vi "Load and Save Example.vi"() -> ()   [LabVIEW 2015]
uses:
  poly_persist_controls_auto_read.vi
  core_persist_controls_auto.vi
  poly_persist_controls_auto_write.vi
panel:
  in  "Cancel":bool
  in  "OK":bool
  in  "Numeric Option 2":dbl
  in  "Numeric Option 1":dbl
  in  "Option 4":bool
  in  "Option 3":bool
  in  "Option 2":bool
  in  "Option 1":bool
  in  "User":u16(ring) items=["John", "Paul", "George", "Ringo"]
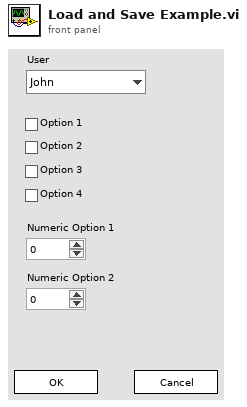
[diagram p1: front panel]
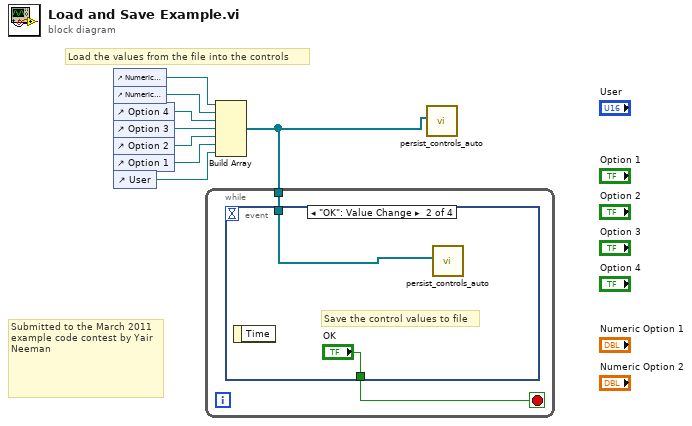
[diagram p0: block diagram]
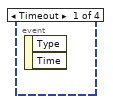
[diagram p2: hidden frame]
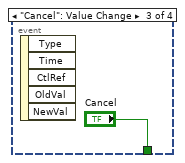
[diagram p3: hidden frame]
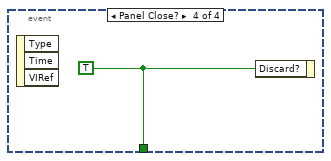
[diagram p4: hidden frame]
diagram:
  # "Submitted to the March 2011 example code contest by Yair Neeman"
  # "Load the values from the file into the controls"
  n1 = control-ref of="Numeric Option 2"() -> (w8:refnum<vi>)
  n2 = control-ref of="Numeric Option 1"() -> (w7:refnum<vi>)
  n3 = control-ref of="Option 4"() -> (w6:refnum<vi>)
  n4 = control-ref of="Option 3"() -> (w5:refnum<vi>)
  n5 = control-ref of="Option 2"() -> (w4:refnum<vi>)
  n6 = control-ref of="Option 1"() -> (w3:refnum<vi>)
  n7 = control-ref of="User"() -> (w2:refnum<vi>)
  n8 = Build Array(w8, w7, w6, w5, w4, w3, w2) -> (w1:refnum<vi>[])
  n9 = while {
    tunnel: w1 -> [w9]
    stop <- w10 stop-if-true
    n10 = event shown="[1] \"OK\": Value Change" {
      selector: _ -> [_ _ _ _]
      dyn-events: _ -> [_ _ _ _]
      timeout: _ -> [_ _ _ _]
      tunnel: [_ "OK" "Cancel" w14] -> w10
      tunnel: w9 -> [_ w11 _ _]
      event Timeout {
        n11 = event-data() -> ()  [unwired: 1 in, 2 out]
      }
      event "OK": Value Change {
        # "Save the control values to file"
        n12 = event-data() -> ()  [unwired: 1 in, 1 out]
        n13 = call-poly "persist_controls_auto.vi"("ctrl refs in"=w11) -> ()  [unwired: 9 in, 2 out]
      }
      event "Cancel": Value Change {
        n14 = event-data() -> ()  [unwired: 1 in, 5 out]
      }
      event Panel Close? {
        w14 = TRUE
        n15 = event-data() -> ()  [unwired: 1 in, 3 out]
        n16 = event-data("Discard?"=w14) -> ()  [unwired: 1 in, 1 out]
      }
    }
  }
  n17 = call-poly "persist_controls_auto.vi"("ctrl refs in"=w1) -> ()  [unwired: 9 in, 2 out]
